vi "缓起(子VI).vi"(7 "循环数(100)":dbl=100.0 format="%#_13g", 10 "缓起清零":bool, 11 "输入":variant) -> (3 "输出":i32[](array[numeric]))   [LabVIEW 2017]
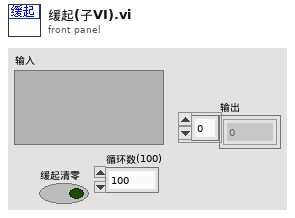
[diagram p1: front panel]
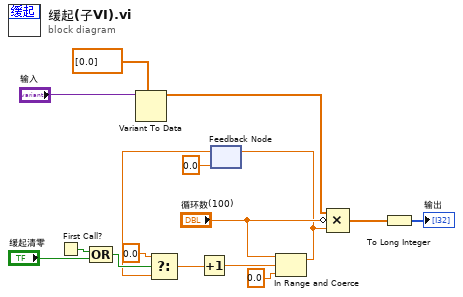
[diagram p0: block diagram]
diagram:
  n1 = First Call?() -> (First Call?: T/F=w9:bool)
  n2 = Compound Arithmetic op=OR ("复合运算")(w9, "缓起清零") -> (w14:bool)
  n3 = Variant To Data(type=dbl[] [0.0], Variant="输入") -> (data=w1:dbl[])  [unwired: 1 in, 1 out]
  n4 = feedback #1(0.0) -> (w8:dbl)
  n5 = Select(t=0.0, s=w14, f=w8) -> (s? t:f=w11:dbl)
  n6 = Increment(x=w11) -> (x+1=w6:dbl)
  n7 = In Range and Coerce(upper limit="循环数(100)", x=w6, lower limit=0.0 ("下限")) -> (coerced(x)=w12:dbl)  [unwired: 1 out]
  n8 = feedback-in #1(w12) -> ()
  n9 = Compound Arithmetic op=MULTIPLY(w1, invert "循环数(100)", w12) -> (w16:dbl[])
  n10 = To Long Integer(number=w16) -> (32bit integer=→"输出":i32[])
